vi "Collect Data Stop.vi"(8 "error in (no error)":errorcluster) -> (0 "error out":errorcluster)   [LabVIEW 2015, in "Tool Interface.lvlib"]
uses:
  Tool Interface.lvlib
  Tool Typedefs/_Collect Data Params Cluster--typedef.ctl
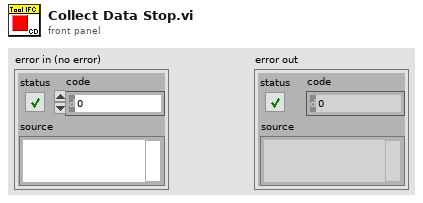
[diagram p1: front panel]
types:
  T1 = typedef "_Collect Data Params Cluster--typedef.ctl" = cluster{"Start":bool, "Immediate":bool, "Lasers ON?":bool, "Length":i32}
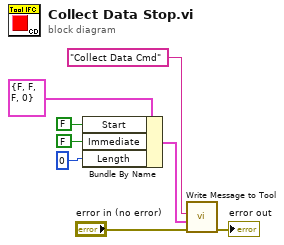
[diagram p0: block diagram]
diagram:
  n1 = Bundle By Name(cluster=T1 {"Start"=FALSE, "Immediate"=FALSE, "Lasers ON?"=FALSE, "Length"=0} ("_Laser Params Cluster--typedef"), "Start"=FALSE, "Immediate"=FALSE, "Length"=0) -> (w7:T1)
  n2 = call "Write Message to Tool.vi"("error in (no error)"="error in (no error)", "Message Data"=w7, "Message"="Collect Data Cmd") -> ("error out"=→"error out":errorcluster)  [unwired: 8 in]
